vi "Write Multi I8 as Numeric.vi"(8 "error in (no error)":errorcluster, 9 "Array":i8[](array[numeric]), 10 "Tag":string[](array[string]), 11 "Omni_Bus in":refnum<class "Omni_Bus.lvclass">) -> (0 "error out":errorcluster, 3 "Omni_Bus out":refnum<class "Omni_Bus.lvclass">)   [LabVIEW 2021, in "Omni_Bus.lvclass"]
uses:
  Omni_Bus.lvclass
  Omni_Bus.lvclass/Omni_Bus.ctl
  <vilib>/TSA/Abstract Data Classes/Abs_Types/Numeric/Abs_Numeric.lvclass
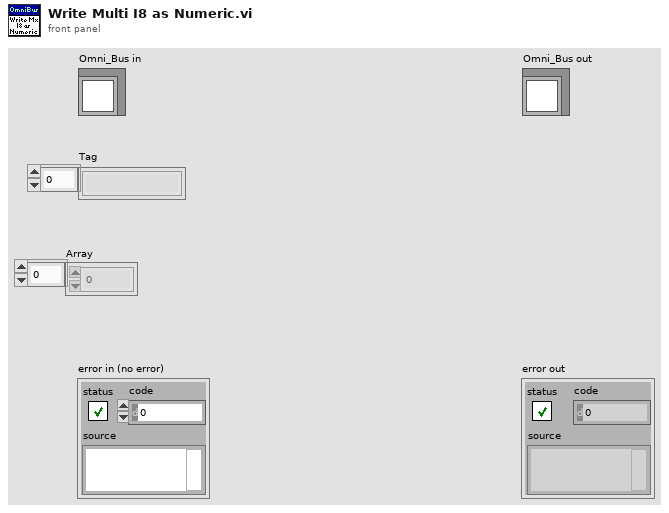
[diagram p1: front panel]
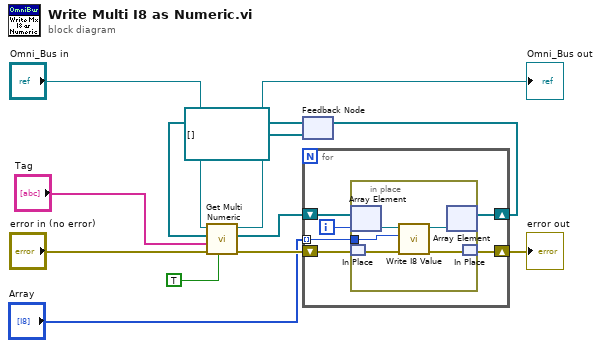
[diagram p0: block diagram]
diagram:
  n1 = feedback #1(refnum<class "Abs_Numeric.lvclass">[] []) -> (w8:refnum<class "Abs_Numeric.lvclass">[])
  n2 = call-dynamic "Get Multi Numeric.vi"("Write?"=TRUE, "error in (no error)"="error in (no error)", "Tag"="Tag", "Value Type"=w8, "Var Bus in"="Omni_Bus in") -> ("error out"=w5:errorcluster, "Value Out"=w4:refnum<class "Abs_Numeric.lvclass">[], "Var Bus out"=→"Omni_Bus out":refnum<class "Omni_Bus.lvclass">)  [unwired: 4 in]
  n3 = for {
    tunnel: "Array" -> [w18] mode=indexing
    shift-right: [w13] -> w2
    shift-left: w5 -> [w14]
    shift-right: [w16] -> w1
    shift-left: w4 -> [w17]
    i -> [w15]
    n4 = in-place {
      in-place-border: w18 -> [w23]
      n5 = in-place-array #2(w17, w15) -> (w22:refnum<class "Abs_Numeric.lvclass">)
      n6 = in-place-match #3(w14) -> (w20:errorcluster)
      n7 = call-dynamic "Write I8 Value.vi"("error in (no error)"=w20, "I8"=w23, "Numeric in"=w22) -> ("error out"=w19:errorcluster, "Numeric out"=w21:refnum<class "Abs_Numeric.lvclass">)  [unwired: 7 in]
      n8 = in-place-array #2(w21) -> (w16:refnum<class "Abs_Numeric.lvclass">[])  [unwired: 1 out]
      n9 = in-place-match #3(w19) -> (w13:errorcluster)
    }
  }
  "error out" <- w2
  n10 = feedback-in #1(w1) -> ()
